vi "Insert New Num.vi"(11 "board in":dbl[][](array[numeric])) -> (3 "board out":dbl[][](array[numeric]))   [LabVIEW 2015]
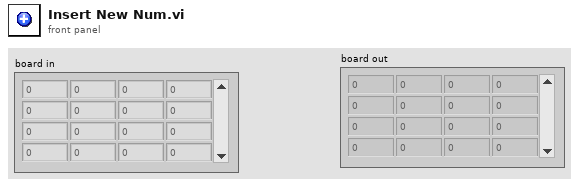
[diagram p1: front panel]
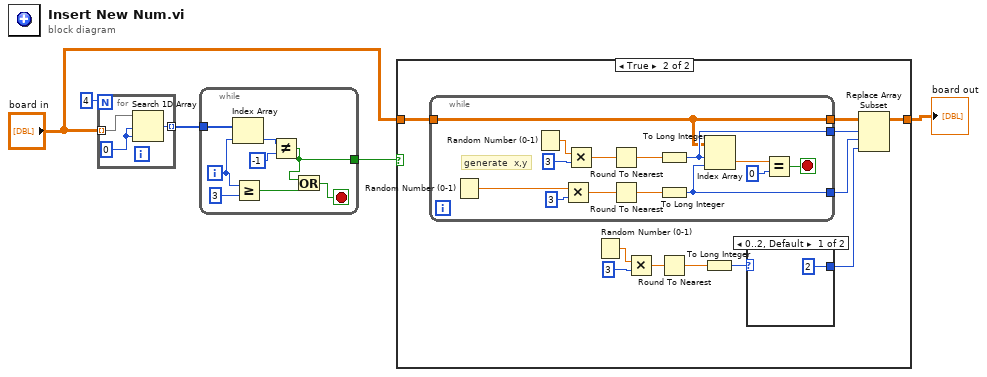
[diagram p0: block diagram]
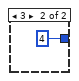
[diagram p3: hidden frame]
diagram:
  n1 = for {
    N: 4 -> [_]
    tunnel: "board in" -> [w8] mode=indexing
    tunnel: [w6] -> w3 mode=indexing
    w7 = 0
    n2 = Search 1D Array(1D array=w8, element=w7, start index (0)=w7) -> (index of element=w6:i32)
  }
  n3 = while {
    tunnel: w3 -> [w13]
    tunnel: [w9] -> w2
    i -> [w12]
    stop <- w14 stop-if-true
    n4 = Index Array(array=w13, index=w12) -> (element=w11:i32)
    n5 = Greater Or Equal?(x=w12, y=3) -> (x >= y?=w15:bool)
    n6 = Not Equal?(x=w11, y=-1) -> (x != y?=w9:bool)
    n7 = Or(x=w9, y=w15) -> (x .or. y?=w14:bool)
  }
  n8 = case shown="True" w2 {
    tunnel: [w17 w19] -> w5
    tunnel: "board in" -> [w17 w18]
    frame False {
    }
    frame True {
      n9 = while {
        tunnel: w18 -> [w29]
        tunnel: [w31] -> w22
        tunnel: [w30] -> w21
        tunnel: [w29] -> w23
        stop <- w40 stop-if-true
        # "generate  x,y"
        n10 = Random Number (0-1)() -> (number: 0 to 1=w36:dbl)
        n11 = Random Number (0-1)() -> (number: 0 to 1=w39:dbl)
        n12 = Multiply(x=w36, y=3) -> (x*y=w33:dbl)
        n13 = Multiply(x=w39, y=3) -> (x*y=w35:dbl)
        n14 = Round To Nearest(number=w35) -> (nearest integer value=w34:dbl)
        n15 = Round To Nearest(number=w33) -> (nearest integer value=w32:dbl)
        n16 = To Long Integer(number=w34) -> (32bit integer=w31:i32)
        n17 = To Long Integer(number=w32) -> (32bit integer=w30:i32)
        n18 = Index Array(array=w29, index (row)=w31, index (col)=w30) -> (element=w42:dbl)
        n19 = Equal?(x=w42, y=0) -> (x = y?=w40:bool)
      }
      n20 = Random Number (0-1)() -> (number: 0 to 1=w27:dbl)
      n21 = Multiply(x=w27, y=3) -> (x*y=w26:dbl)
      n22 = Round To Nearest(number=w26) -> (nearest integer value=w25:dbl)
      n23 = To Long Integer(number=w25) -> (32bit integer=w24:i32)
      n24 = case shown="0..2, Default" w24 {
        tunnel: [2 4] -> w20
        frame 0..2, Default {
        }
        frame 3 {
        }
      }
      n25 = Replace Array Subset(array=w23, new element=w20, index (row)=w22, index (col)=w21) -> (w19:dbl[][])
    }
  }
  "board out" <- w5
